vi "AE_VALVE_CONTROL.vi"(7 "Action":enum16{"Set", "Set All", "Get", "Get All"}(ring), 8 "Array In":bool[](array[boolean]), 9 "Bool In":bool, 10 "Channel ID":i32=-999999, 11 "DAQmx Global Channel":refnum<k21>="AIR_BLEED") -> (2 "All Channel Status":bool[](array[boolean]), 3 "Selected Status":bool)   [LabVIEW 2013]
doc: "An action engine for controlling the valves. Can set and get states for either a specific valve or all."
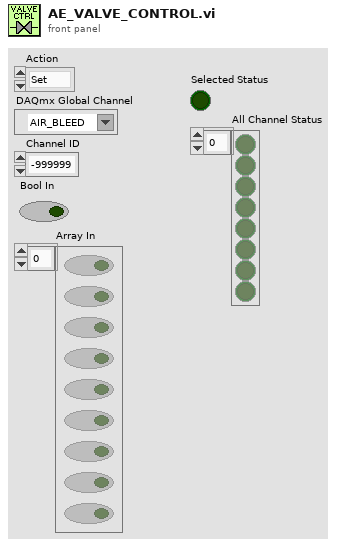
[diagram p1: front panel]
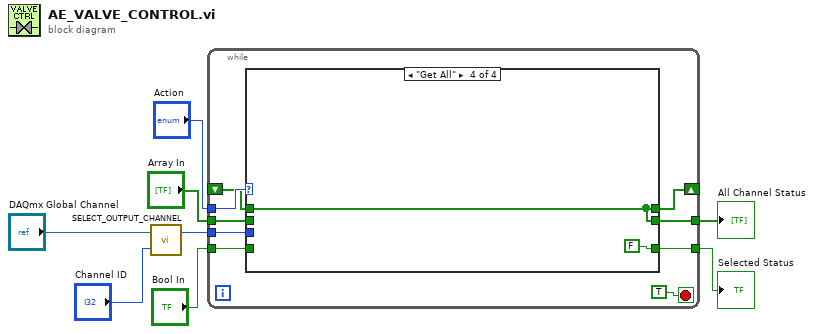
[diagram p0: block diagram]
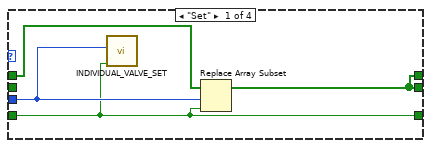
[diagram p2: hidden frame]
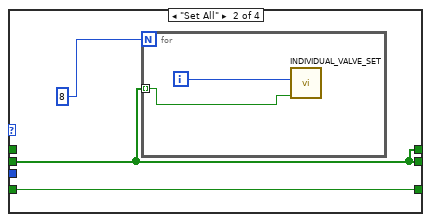
[diagram p3: hidden frame]
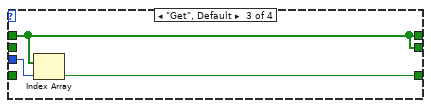
[diagram p4: hidden frame]
diagram:
  n1 = call "SELECT_OUTPUT_CHANNEL.vi"("Channel ID IN"="Channel ID", "DAQmx Global Channel IN"="DAQmx Global Channel") -> ("Channel ID OUT"=w3:i32)  [unwired: 1 out]
  n2 = while {
    tunnel: "Action" -> [w16]
    shift-right: [w9] -> _
    shift-left: _ -> [w15]
    tunnel: "Bool In" -> [w14]
    tunnel: "Array In" -> [w12]
    tunnel: w3 -> [w13]
    tunnel: [w11] -> w2
    tunnel: [w10] -> w1
    stop <- TRUE stop-if-true
    n3 = case shown="\"Get All\"" w16 {
      tunnel: w15 -> [w21 _ w27 w30]
      tunnel: w14 -> [w18 w24 _ _]
      tunnel: w13 -> [w19 _ w29 _]
      tunnel: w12 -> [_ w23 _ _]
      tunnel: [w20 w23 w27 w30] -> w11
      tunnel: [w18 w24 w28 FALSE] -> w10
      tunnel: [w20 w23 w27 w30] -> w9
      frame "Set" {
        n4 = call "INDIVIDUAL_VALVE_SET.vi"("Input Value"=w18, "Channel ID IN"=w19) -> ()  [unwired: 10 in]
        n5 = Replace Array Subset(array=w21, new element=w18, index=w19) -> (w20:bool[])
      }
      frame "Set All" {
        n6 = for {
          N: 8 -> [_]
          tunnel: w23 -> [w26] mode=indexing
          i -> [w25]
          n7 = call "INDIVIDUAL_VALVE_SET.vi"("Input Value"=w26, "Channel ID IN"=w25) -> ()  [unwired: 10 in]
        }
      }
      frame "Get", Default {
        n8 = Index Array(array=w27, index=w29) -> (element=w28:bool)
      }
      frame "Get All" {
      }
    }
  }
  "Selected Status" <- w1
  "All Channel Status" <- w2
